vi "create header.vi"(11 "unique key":string) -> (3 "wire data":string)   [LabVIEW 2013, in "TEC runtime.lvclass"]
uses:
  TEC runtime.lvclass
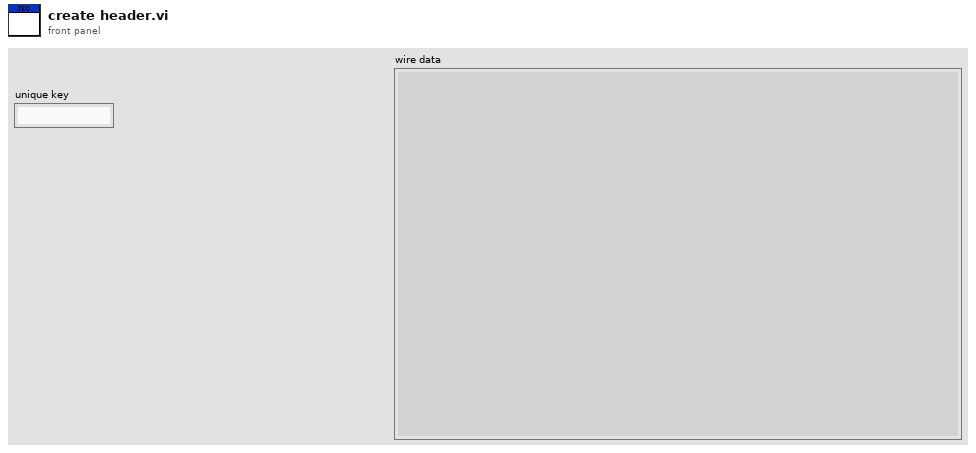
[diagram p1: front panel]
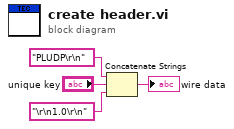
[diagram p0: block diagram]
diagram:
  n1 = Concatenate Strings("PLUDP\r\n" ("string"), "unique key", "\r\n1.0\r\n" ("string")) -> (→"wire data":string)
